vi "IMU data.vi"(0 "stop 4":bool, 1 "milliseconds to wait 2":u32, 5 "milliseconds to wait 4":u32, 7 "milliseconds to wait":u32, 9 "stop 5":bool, 12 "stop in":bool) -> (3 "?":dbl, 4 "Y 2":i16, 6 "Z 2":i16, 8 "X 2":i16, 10 "Z":i16, 13 "X":i16, 14 "Y":i16)   [LabVIEW 2013]
uses:
  <vilib>/LabVIEW Interface for Arduino/Type Defs/Board Type.ctl
  <vilib>/LabVIEW Interface for Arduino/Type Defs/Connection Type.ctl
  <vilib>/LabVIEW Interface for Arduino/LabVIEW Interface for Arduino.lvlib
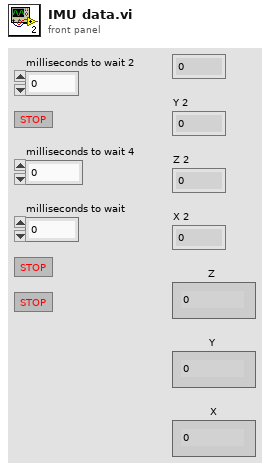
[diagram p1: front panel]
types:
  T1 = typedef "LabVIEW Interface for Arduino.lvlib/Connection Type.ctl" = enum8{"USB / Serial", "XBEE", "BlueSmirf (Bluetooth)"}
  T2 = typedef "LabVIEW Interface for Arduino.lvlib/Board Type.ctl" = enum16{"Uno", "Dimuelanove w/Atmega 328", "Mega 2560"}
  T3 = typedef "LabVIEW Interface for Arduino.lvlib/Arduino Resource.ctl" = cluster{"VISA resource":refnum<visa-resource-name>, "Board Type":T2, "Connection Type":enum8{"USB / Serial"}, "Bytes Per Packet (15)":u8}
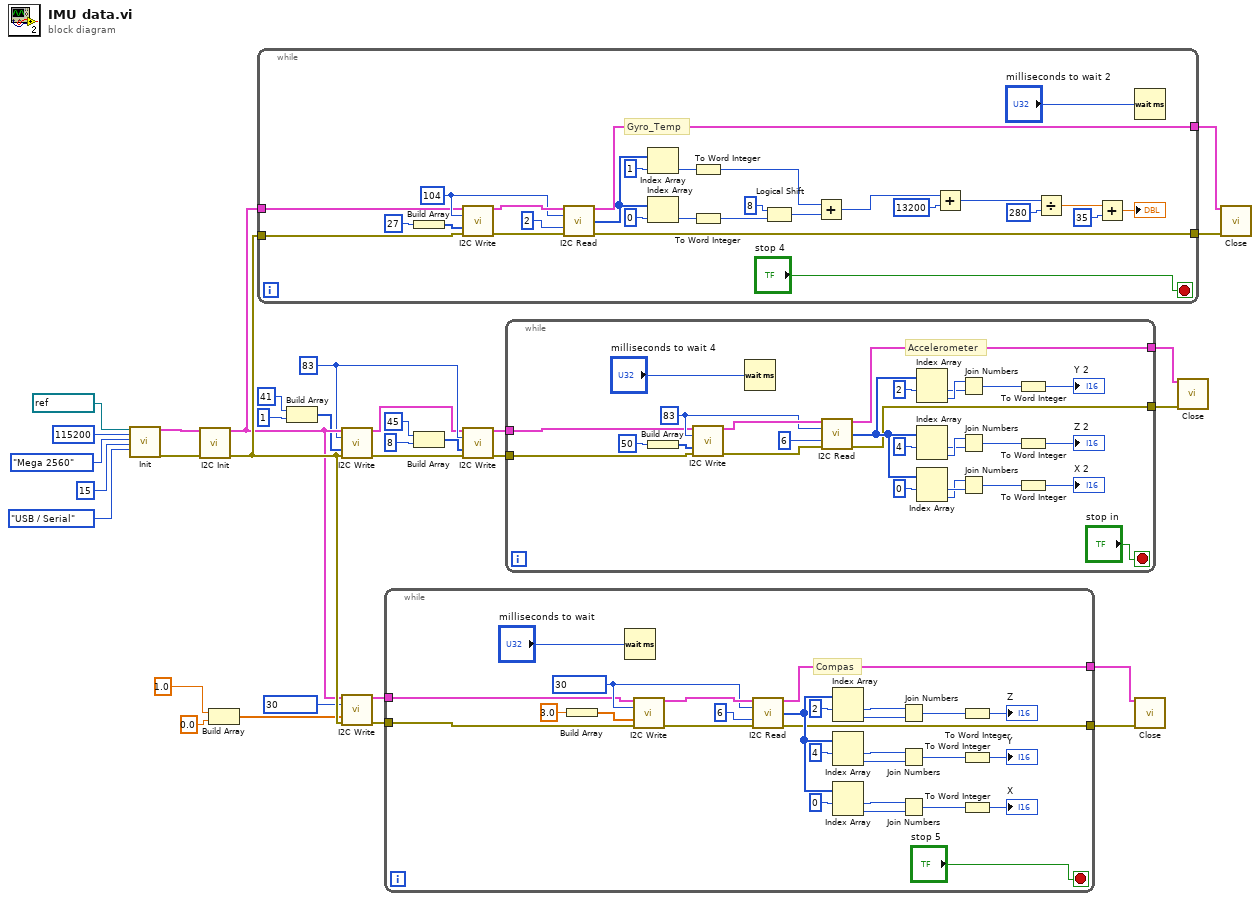
[diagram p0: block diagram]
diagram:
  w13 = u8 83 ("Address (0)")
  n1 = call <vilib>:"Init.vi"("VISA resource"=refnum<visa-resource-name> "COM4", "Baud Rate (115200)"=u32 115200, "Board Type (Uno)"=Board_Type."Mega 2560", "Bytes Per Packet (15)"=u32 15, "Connection Type (USB/Serial)"=Connection_Type."USB / Serial") -> ("Arduino Resource"=w3:T3, "error out"=w4:errorcluster)  [unwired: 13 in]
  n2 = call <vilib>:"I2C Init.vi"("Arduino Resource"=w3, "error in"=w4) -> ("Arduino Resource"=w27:T3, "error out"=w28:errorcluster)  [unwired: 12 in]
  n3 = Build Array(1.0 ("element"), 0.0 ("element")) -> (w19:dbl[])
  n4 = while {
    tunnel: [w38] -> w16
    tunnel: [w37] -> w17
    tunnel: w27 -> [w36]
    tunnel: w28 -> [w35]
    stop <- "stop 4" stop-if-true
    w58 = u8 104 ("Address (0)")
    # "Gyro_Temp"
    n5 = Build Array(u8 27 ("Bytes To Read")) -> (w55:u8[])
    n6 = call <vilib>:"I2C Write.vi"("Arduino Resource"=w36, "Address (0)"=w58, "I2C Data Bytes"=w55, "error in"=w35) -> ("Arduino Resource"=w60:T3, "error out"=w59:errorcluster)  [unwired: 10 in]
    n7 = call <vilib>:"I2C Read.vi"("Arduino Resource"=w60, "Address (0)"=w58, "Bytes To Read"=u8 2, "error in"=w59) -> ("Arduino Resource"=w38:T3, "I2C Data"=w42:u8[], "error out"=w37:errorcluster)  [unwired: 9 in]
    n8 = Index Array(array=w42, index=u8 1) -> (element=w41:u8)
    n9 = Index Array(array=w42, index=u8 0) -> (element=w40:u8)
    n10 = To Word Integer(number=w41) -> (16bit integer=w53:i16)
    n11 = To Word Integer(number=w40) -> (16bit integer=w39:i16)
    n12 = Logical Shift(y=u8 8, x=w39) -> (x << y=w52:i16)
    n13 = Add(x=w53, y=w52) -> (x+y=w47:i16)
    n14 = Add(x=w47, y=i16 13200) -> (x+y=w46:i16)
    n15 = Divide(x=w46, y=i16 280) -> (x/y=w44:dbl)
    n16 = Add(x=w44, y=i16 35) -> (x+y=→"?":dbl)
    n17 = Wait (ms)(milliseconds to wait="milliseconds to wait 2") -> ()  [unwired: 1 out]
  }
  n18 = Build Array(41, 1) -> (w7:i32[])
  n19 = call <vilib>:"I2C Write.vi"("Arduino Resource"=w27, "Address (0)"=w13, "I2C Data Bytes"=w7, "error in"=w28) -> ("Arduino Resource"=w5:T3, "error out"=w6:errorcluster)  [unwired: 10 in]
  n20 = call <vilib>:"I2C Write.vi"("Arduino Resource"=w27, "Address (0)"=u8 30, "I2C Data Bytes"=w19, "error in"=w28) -> ("Arduino Resource"=w23:T3, "error out"=w24:errorcluster)  [unwired: 10 in]
  n21 = while {
    tunnel: [w68] -> w21
    tunnel: [w67] -> w22
    tunnel: w23 -> [w66]
    tunnel: w24 -> [w65]
    stop <- "stop 5" stop-if-true
    w70 = u8 30
    # "Compas"
    n22 = Build Array(3.0 ("element")) -> (w71:dbl[])
    n23 = Wait (ms)(milliseconds to wait="milliseconds to wait") -> ()  [unwired: 1 out]
    n24 = call <vilib>:"I2C Write.vi"("Arduino Resource"=w66, "Address (0)"=w70, "I2C Data Bytes"=w71, "error in"=w65) -> ("Arduino Resource"=w73:T3, "error out"=w72:errorcluster)  [unwired: 10 in]
    n25 = call <vilib>:"I2C Read.vi"("Arduino Resource"=w73, "Address (0)"=w70, "Bytes To Read"=u8 6, "error in"=w72) -> ("Arduino Resource"=w68:T3, "I2C Data"=w83:u8[], "error out"=w67:errorcluster)  [unwired: 9 in]
    n26 = Index Array(array=w83, index #1=2 ("index")) -> (element #1=w79:u8, element #2=w80:u8)  [unwired: 1 in]
    n27 = Index Array(array=w83, index #1=4 ("index")) -> (element #1=w81:u8, element #2=w82:u8)  [unwired: 1 in]
    n28 = Index Array(array=w83, index #1=0 ("index")) -> (element #1=w78:u8, element #2=w77:u8)  [unwired: 1 in]
    n29 = Join Numbers(hi=w79, lo=w80) -> ((hi.lo)=w86:u16)
    n30 = Join Numbers(hi=w81, lo=w82) -> ((hi.lo)=w88:u16)
    n31 = Join Numbers(hi=w78, lo=w77) -> ((hi.lo)=w85:u16)
    n32 = To Word Integer(number=w86) -> (16bit integer=→"Z":i16)
    n33 = To Word Integer(number=w88) -> (16bit integer=→"Y":i16)
    n34 = To Word Integer(number=w85) -> (16bit integer=→"X":i16)
  }
  n35 = Build Array(45, 8) -> (w11:i32[])
  n36 = call <vilib>:"I2C Write.vi"("Arduino Resource"=w5, "Address (0)"=w13, "I2C Data Bytes"=w11, "error in"=w6) -> ("Arduino Resource"=w25:T3, "error out"=w26:errorcluster)  [unwired: 10 in]
  n37 = while {
    tunnel: [w97] -> w14
    tunnel: [w96] -> w15
    tunnel: w25 -> [w95]
    tunnel: w26 -> [w94]
    stop <- "stop in" stop-if-true
    w98 = u8 83 ("Address (0)")
    # "Accelerometer"
    n38 = Build Array(u8 50 ("Bytes To Read")) -> (w112:u8[])
    n39 = call <vilib>:"I2C Write.vi"("Arduino Resource"=w95, "Address (0)"=w98, "I2C Data Bytes"=w112, "error in"=w94) -> ("Arduino Resource"=w116:T3, "error out"=w115:errorcluster)  [unwired: 10 in]
    n40 = Wait (ms)(milliseconds to wait="milliseconds to wait 4") -> ()  [unwired: 1 out]
    n41 = call <vilib>:"I2C Read.vi"("Arduino Resource"=w116, "Address (0)"=w98, "Bytes To Read"=u8 6, "error in"=w115) -> ("Arduino Resource"=w97:T3, "I2C Data"=w99:u8[], "error out"=w96:errorcluster)  [unwired: 9 in]
    n42 = Index Array(array=w99, index #1=2 ("index")) -> (element #1=w105:u8, element #2=w106:u8)  [unwired: 1 in]
    n43 = Index Array(array=w99, index #1=4 ("index")) -> (element #1=w107:u8, element #2=w108:u8)  [unwired: 1 in]
    n44 = Index Array(array=w99, index #1=0 ("index")) -> (element #1=w104:u8, element #2=w103:u8)  [unwired: 1 in]
    n45 = Join Numbers(hi=w106, lo=w105) -> ((hi.lo)=w110:u16)
    n46 = Join Numbers(hi=w108, lo=w107) -> ((hi.lo)=w111:u16)
    n47 = Join Numbers(hi=w103, lo=w104) -> ((hi.lo)=w109:u16)
    n48 = To Word Integer(number=w110) -> (16bit integer=→"Y 2":i16)
    n49 = To Word Integer(number=w111) -> (16bit integer=→"Z 2":i16)
    n50 = To Word Integer(number=w109) -> (16bit integer=→"X 2":i16)
  }
  n51 = call <vilib>:"Close.vi"("Arduino Resource"=w21, "error in"=w22) -> ()  [unwired: 13 in, 1 out]
  n52 = call <vilib>:"Close.vi"("Arduino Resource"=w14, "error in"=w15) -> ()  [unwired: 13 in, 1 out]
  n53 = call <vilib>:"Close.vi"("Arduino Resource"=w16, "error in"=w17) -> ()  [unwired: 13 in, 1 out]
